vi "Open Dev.vi"(8 "error in (no error)":errorcluster, 11 "idxDev":i32=-1) -> (0 "error out":errorcluster, 2 "function return":i32, 3 "hdwf":i32)   [LabVIEW 2014, in "AnalogDiscSDKLv.lvlib"]
doc: "extern \"C\" __declspec(dllexport) int Open_DevLv(int idxDev, HDWF *hdwf);"
uses:
  <instrlib>/AnalogDiscSDKLv/AnalogDiscSDKLv.lvlib
  <instrlib>/AnalogDiscSDKLv/AnalogDiscSDKLv.dll
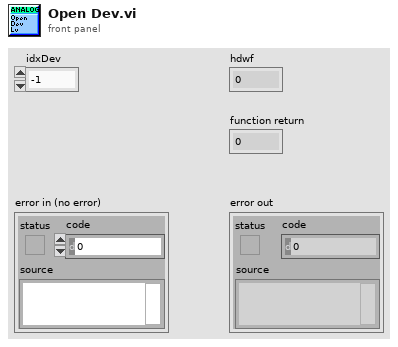
[diagram p1: front panel]
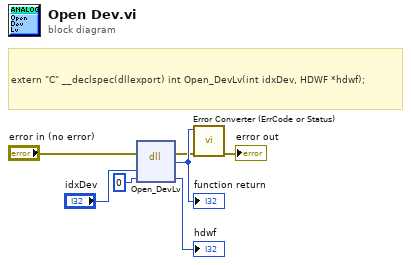
[diagram p0: block diagram]
diagram:
  # "extern \"C\" __declspec(dllexport) int Open_DevLv(int idxDev, HDWF *hdwf);"
  n1 = dll-call lib="C:/Program Files (x86)/National Instruments/LabVIEW 2014/instr.lib/AnalogDiscSDKLv/AnalogDiscSDKLv.*" fn="Open_DevLv"(error in="error in (no error)", "idxDev"="idxDev", "hdwf"=0) -> (error out=w2:errorcluster, w7:i32, "hdwf"=→"hdwf":i32)  [unwired: 3 in, 1 out]
  "function return" <- w7
  n2 = call <instrlib>:"Error Converter (ErrCode or Status).vi"("error in (no error)"=w2, "error code"=w7) -> ("error out"=→"error out":errorcluster)  [unwired: 9 in]
